vi "NI_FPGA_PPG.ProcCases.vi"(0 "i ref in":refnum<vi>, 1 "selector":string, 2 "Data":T1, 3 "call cluster":T2={"Object"="", "Selector"="", "CallType"=enum."synchronous", "Async Object"="", "Async Selector"="", "Data Descriptor"="", "Data"=[], "Error #"=0, "Expire"=0}, 5 "error in (no error)":errorcluster) -> (14 "i ref out":refnum<vi>, 17 "answer cluster":T2={"Object"="", "Selector"="", "CallType"=enum."synchronous", "Async Object"="", "Async Selector"="", "Data Descriptor"="", "Data"=[], "Error #"=0, "Expire"=0}, 19 "error out":errorcluster)   [LabVIEW 2014, in "NI_FPGA_PPG.lvlib"]
doc: "This method is called by a process from within the default case in the event loop. The methods of a class that are linked to events will be called from THIS method. Add your code here."
uses:
  NI_FPGA_PPG.lvlib
  CSCore/CSSystem/CoreDefs/CoreDefs.call_type.ctl
  CSCore/BaseProcess/BaseProcess.descriptor string definition.ctl
  CSCore/CSSystem/CoreDefs/CoreDefs.rawDataType.ctl
  CSCore/CSSystem/CoreLib/CoreLib.string 2 byte array.vi
  CSCore/CSSystem/CoreLib/CoreLib.int 2 byte array.vi
  CSCore/CSSystem/CoreLib/CoreLib.byte array 2 string.vi
  CSCore/CSSystem/CoreLib/CoreLib.byte array 2 int.vi
  CSCore/CSSystem/CoreLib/CoreLib.byte array 2 double.vi
  CSCore/CSSystem/CoreLib/CoreLib.lvlib
  CSCore/BaseProcess/BaseProcess.lvlib
  CSCore/CSApplicationBaseClasses/DeviceBase/DeviceBase.lvlib
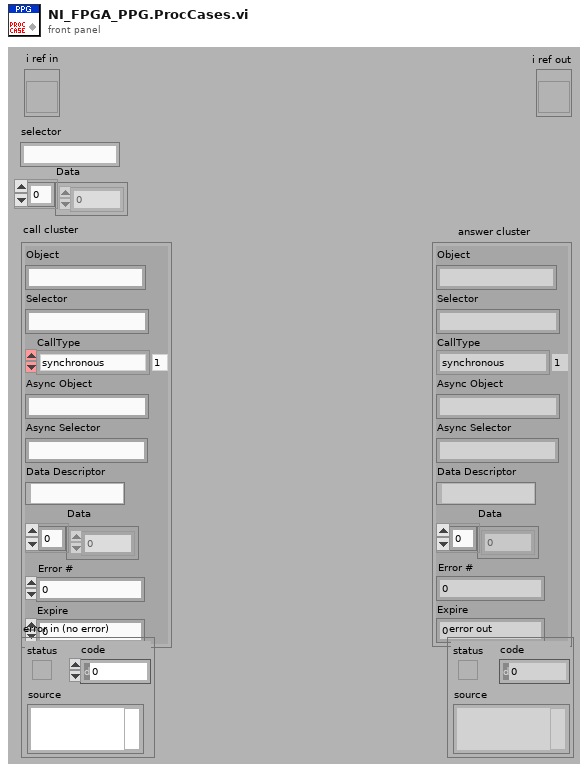
[diagram p1: front panel]
types:
  T1 = typedef "CoreDefs.rawDataType.ctl" = i8[]
  T2 = typedef "CoreDefs.call_type.ctl" = cluster{"Object":string, "Selector":string, "CallType":enum16{"simple", "synchronous", "asynchronous"}, "Async Object":string, "Async Selector":string, "Data Descriptor":T3, "Data":T1, "Error #":i32, "Expire":u32}
  T3 = typedef "BaseProcess.lvlib/BaseProcess.descriptor string definition.ctl" = string
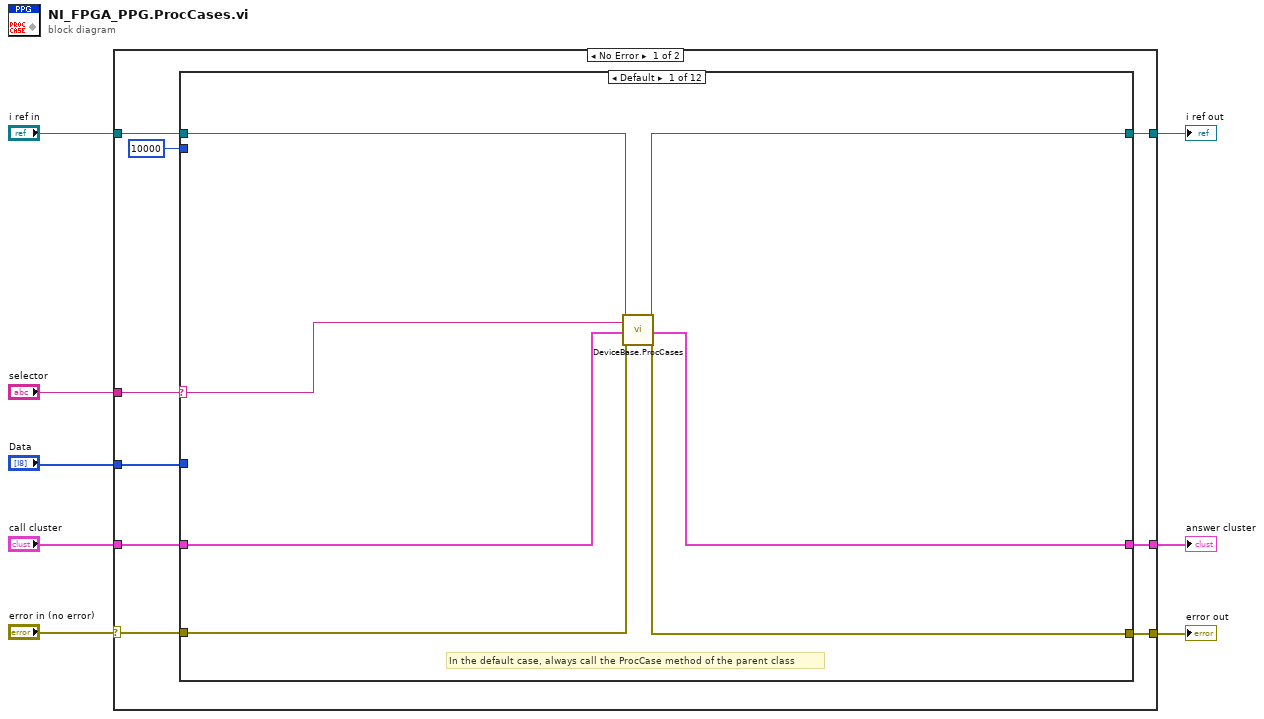
[diagram p0: block diagram]
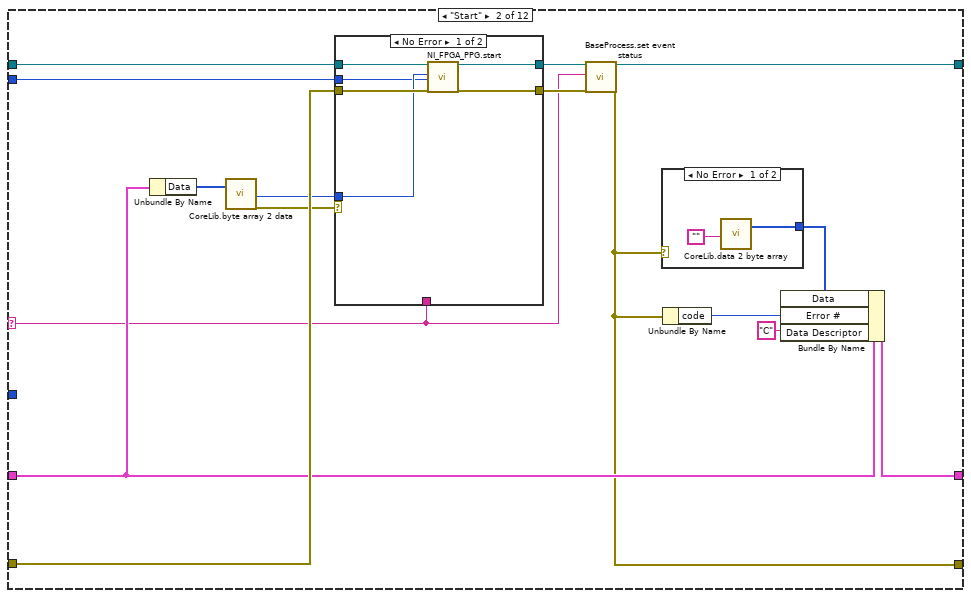
[diagram p2: hidden frame]
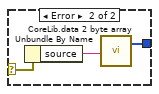
[diagram p3: hidden frame]
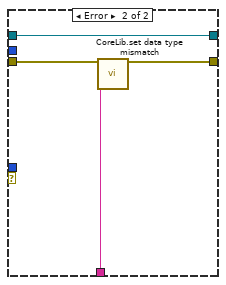
[diagram p4: hidden frame]
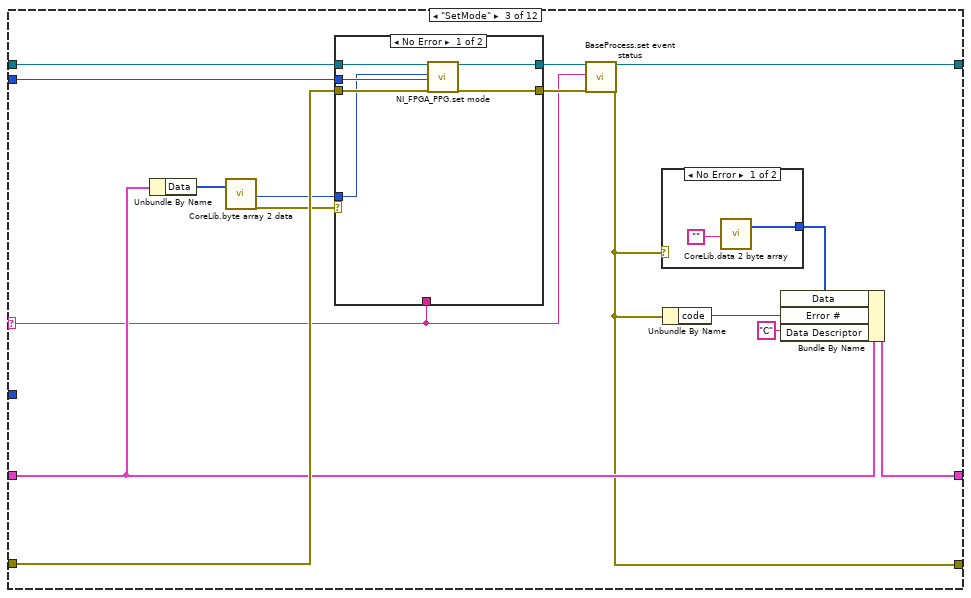
[diagram p5: hidden frame]
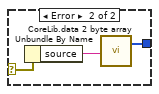
[diagram p6: hidden frame]
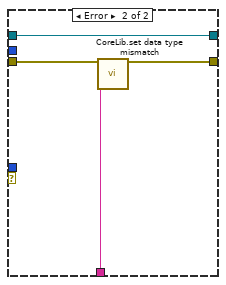
[diagram p7: hidden frame]
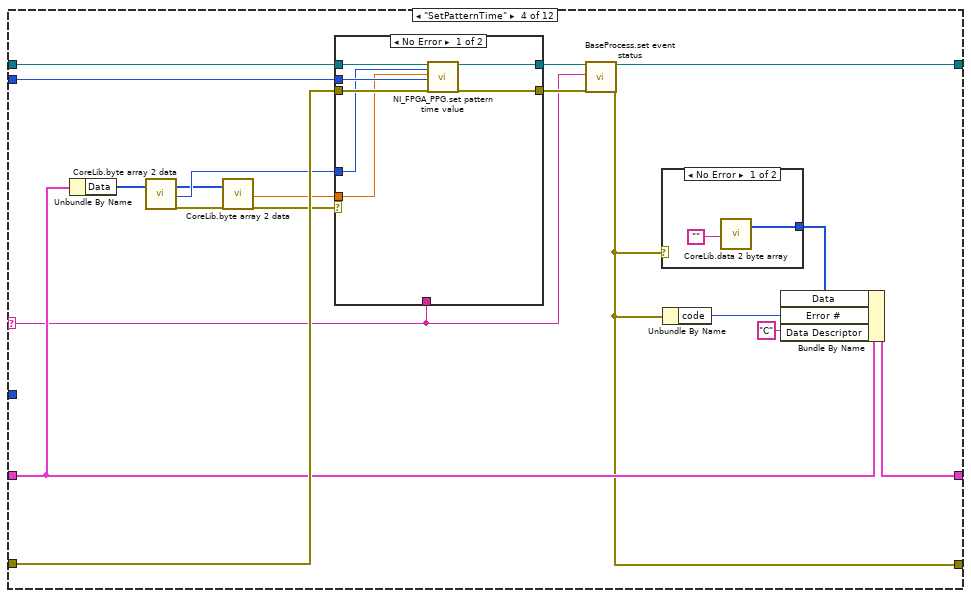
[diagram p8: hidden frame]
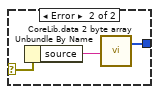
[diagram p9: hidden frame]
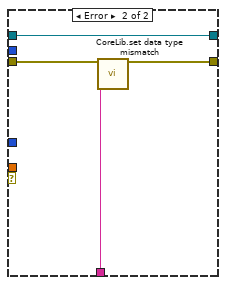
[diagram p10: hidden frame]
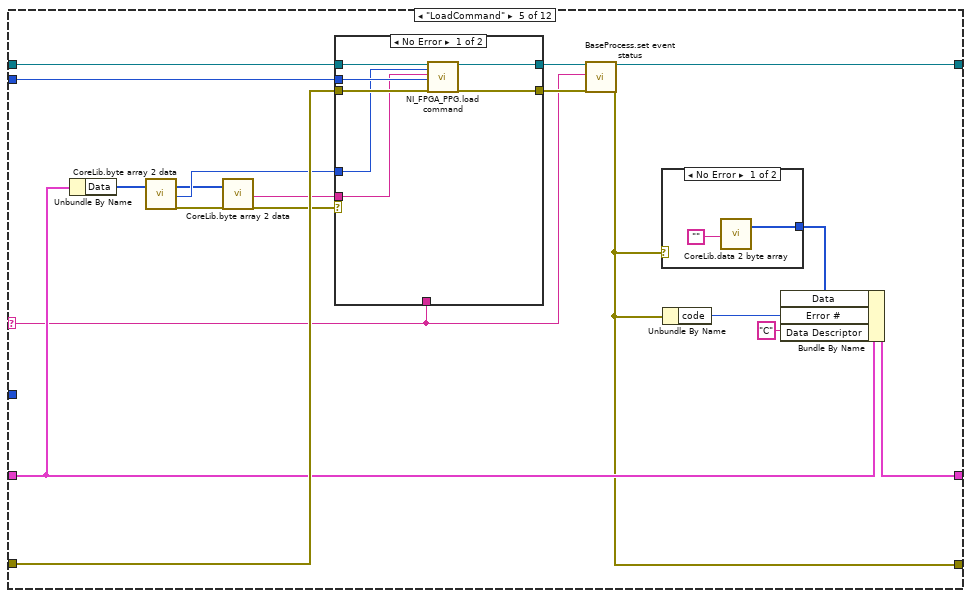
[diagram p11: hidden frame]
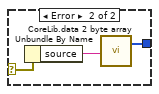
[diagram p12: hidden frame]
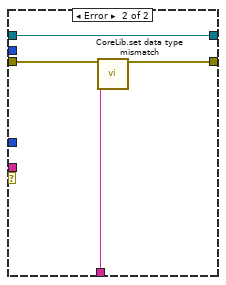
[diagram p13: hidden frame]
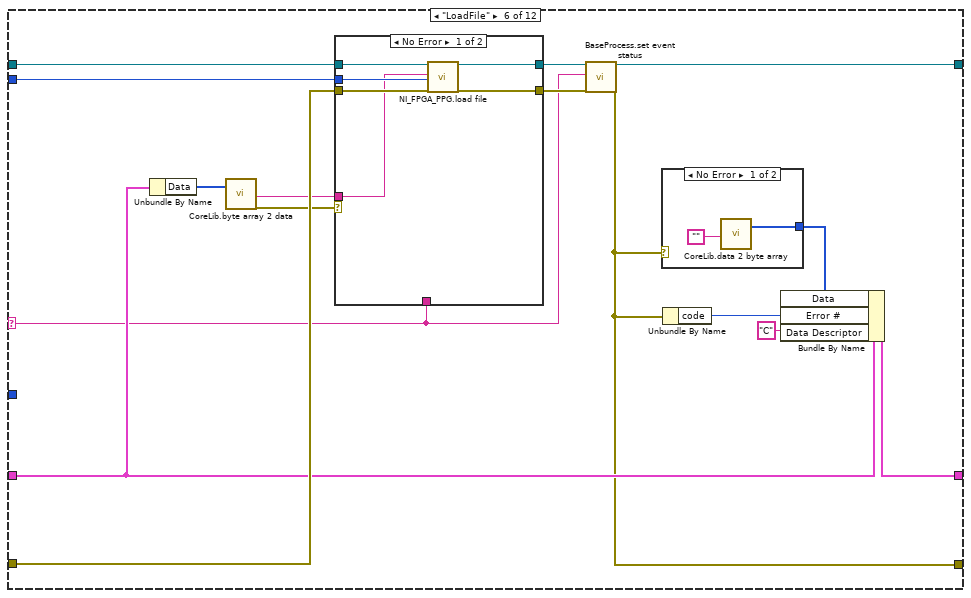
[diagram p14: hidden frame]
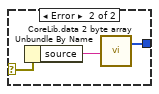
[diagram p15: hidden frame]
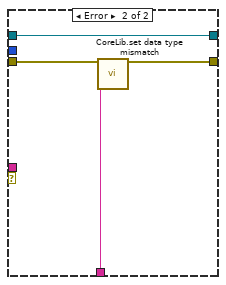
[diagram p16: hidden frame]
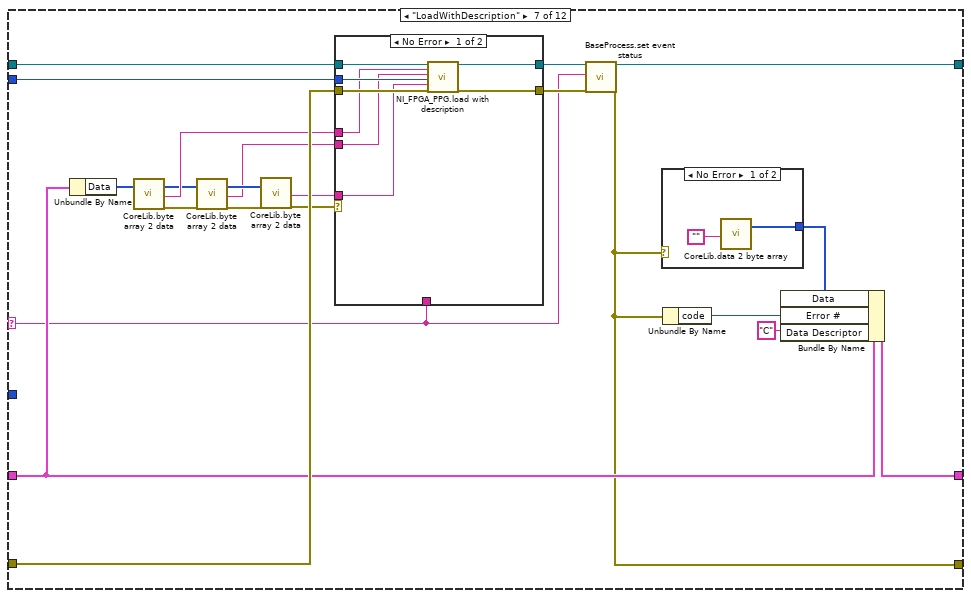
[diagram p17: hidden frame]
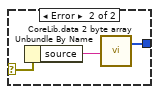
[diagram p18: hidden frame]
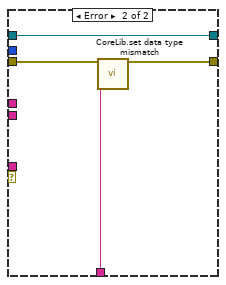
[diagram p19: hidden frame]
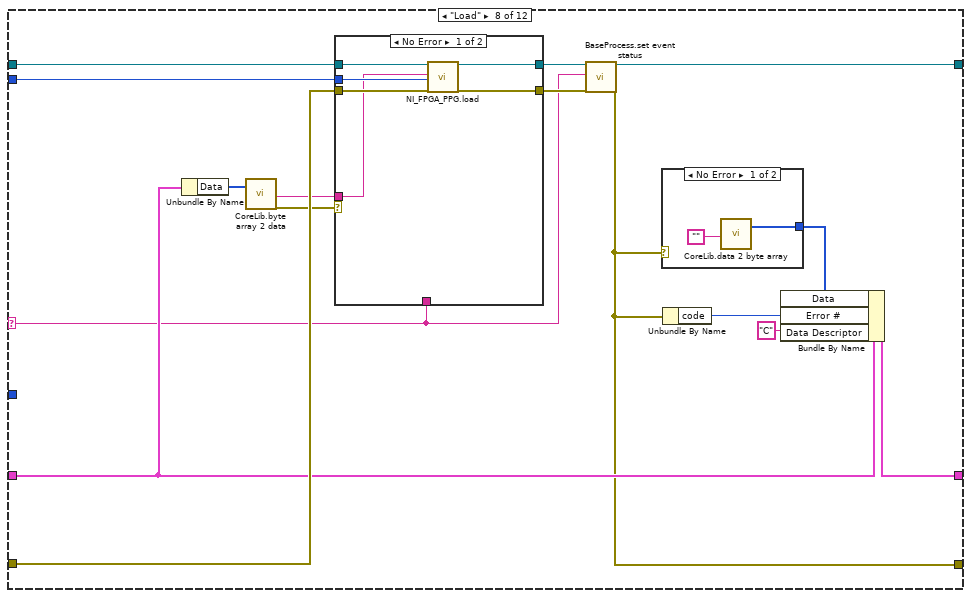
[diagram p20: hidden frame]
diagram:
  n1 = case shown="No Error" "error in (no error)" {
    selector: "error in (no error)" -> [w10 w331]
    tunnel: "selector" -> [w17 _]
    tunnel: [w16 w332] -> w7
    tunnel: "Data" -> [w15 _]
    tunnel: "call cluster" -> [w14 w332]
    tunnel: "i ref in" -> [w13 w333]
    tunnel: [w12 w333] -> w3
    tunnel: [w11 w331] -> w2
    frame No Error {
      n2 = case shown="Default" w17 {
        selector: w17 -> [w19 w31 w62 w96 w131 w163 w200 w233 w261 w279 w298 w316]
        tunnel: w15 -> [_ _ _ _ _ _ _ _ _ _ _ _]
        tunnel: w13 -> [w18 w40 w71 w105 w140 w172 w209 w242 w270 w288 w307 w325]
        tunnel: [w24 w30 w61 w95 w130 w162 w199 w232 w260 w278 w297 w315] -> w12
        tunnel: w14 -> [w20 w37 w68 w102 w137 w169 w206 w239 w267 w285 w304 w322]
        tunnel: [w21 w36 w67 w101 w136 w168 w205 w238 w266 w284 w303 w321] -> w16
        tunnel: w10 -> [w23 w39 w70 w104 w139 w171 w208 w241 w269 w287 w306 w324]
        tunnel: [w22 w32 w63 w97 w132 w164 w201 w234 w262 w280 w299 w317] -> w11
        tunnel: 10000 ("ms timeout") -> [_ w25 w56 w87 w122 w157 w188 w227 w258 w276 w295 w313]
        frame Default {
          # "In the default case, always call the ProcCase method of the parent class"
          n3 = call "DeviceBase.ProcCases.vi"("i ref in"=w18, "selector"=w19, "call cluster"=w20, "error in (no error)"=w23) -> ("i ref out"=w24:refnum<vi>, "answer cluster"=w21:T2, "error out"=w22:errorcluster)  [unwired: 13 in]
        }
        frame "Start" {
          n4 = Unbundle By Name(w37) -> ("Data"=w28:T1)
          n5 = call-poly "CoreLib.byte array 2 data.vi"("byteArray"=w28) -> ("i32"=w27:i32, "error out"=w26:errorcluster)  [unwired: 16 in, 1 out]
          n6 = case shown="No Error" w26 {
            tunnel: [w48 w55] -> w34
            tunnel: w40 -> [w51 w55]
            tunnel: w39 -> [w50 w54]
            tunnel: [w49 w53] -> w33
            tunnel: w31 -> [_ w52]
            tunnel: w27 -> [w47 _]
            tunnel: w25 -> [w46 _]
            frame No Error {
              n7 = call "NI_FPGA_PPG.start.vi"("i ref in"=w51, "start_addr"=w47, "ms timeout (10000)"=w46, "error in (no error)"=w50) -> ("i ref out"=w48:refnum<vi>, "error out"=w49:errorcluster)  [unwired: 13 in, 1 out]
            }
            frame Error {
              n8 = call "CoreLib.set data type mismatch.vi"("error in (no error)"=w54, "error source"=w52) -> ("error out"=w53:errorcluster)  [unwired: 17 in]
            }
          }
          n9 = call "BaseProcess.set event status.vi"("i ref in"=w34, "EventStatus"=w31, "error in (no error)"=w33) -> ("i ref out"=w30:refnum<vi>, "error out"=w32:errorcluster)  [unwired: 14 in, 1 out]
          n10 = case shown="No Error" w32 {
            selector: w32 -> [_ w45]
            tunnel: [w42 w44] -> w35
            frame No Error {
              n11 = call-poly "CoreLib.data 2 byte array.vi"("string"="" ("Empty String Constant")) -> ("byteArray out"=w42:T1)  [unwired: 18 in]
            }
            frame Error {
              n12 = Unbundle By Name(w45) -> ("source"=w43:string)
              n13 = call-poly "CoreLib.data 2 byte array.vi"("string"=w43) -> ("byteArray out"=w44:T1)  [unwired: 18 in]
            }
          }
          n14 = Unbundle By Name(w32) -> ("code"=w38:i32)
          n15 = Bundle By Name(cluster=w37, "Data"=w35, "Error #"=w38, "Data Descriptor"="C") -> (w36:T2)
        }
        frame "SetMode" {
          n16 = Unbundle By Name(w68) -> ("Data"=w59:T1)
          n17 = call-poly "CoreLib.byte array 2 data.vi"("byteArray"=w59) -> ("i32"=w58:i32, "error out"=w57:errorcluster)  [unwired: 16 in, 1 out]
          n18 = case shown="No Error" w57 {
            tunnel: [w79 w86] -> w65
            tunnel: w71 -> [w82 w86]
            tunnel: w70 -> [w81 w85]
            tunnel: [w80 w84] -> w64
            tunnel: w62 -> [_ w83]
            tunnel: w58 -> [w77 _]
            tunnel: w56 -> [w78 _]
            frame No Error {
              n19 = call "NI_FPGA_PPG.set mode.vi"("i ref in"=w82, "mode"=w77, "ms timeout (10000)"=w78, "error in (no error)"=w81) -> ("i ref out"=w79:refnum<vi>, "error out"=w80:errorcluster)  [unwired: 13 in, 1 out]
            }
            frame Error {
              n20 = call "CoreLib.set data type mismatch.vi"("error in (no error)"=w85, "error source"=w83) -> ("error out"=w84:errorcluster)  [unwired: 17 in]
            }
          }
          n21 = call "BaseProcess.set event status.vi"("i ref in"=w65, "EventStatus"=w62, "error in (no error)"=w64) -> ("i ref out"=w61:refnum<vi>, "error out"=w63:errorcluster)  [unwired: 14 in, 1 out]
          n22 = case shown="No Error" w63 {
            selector: w63 -> [_ w76]
            tunnel: [w73 w75] -> w66
            frame No Error {
              n23 = call-poly "CoreLib.data 2 byte array.vi"("string"="" ("Empty String Constant")) -> ("byteArray out"=w73:T1)  [unwired: 18 in]
            }
            frame Error {
              n24 = Unbundle By Name(w76) -> ("source"=w74:string)
              n25 = call-poly "CoreLib.data 2 byte array.vi"("string"=w74) -> ("byteArray out"=w75:T1)  [unwired: 18 in]
            }
          }
          n26 = Unbundle By Name(w63) -> ("code"=w69:i32)
          n27 = Bundle By Name(cluster=w68, "Data"=w66, "Error #"=w69, "Data Descriptor"="C") -> (w67:T2)
        }
        frame "SetPatternTime" {
          n28 = Unbundle By Name(w102) -> ("Data"=w93:T1)
          n29 = call-poly "CoreLib.byte array 2 data.vi"("byteArray"=w93) -> ("byteArray out"=w90:T1, "i32"=w92:i32, "error out"=w91:errorcluster)  [unwired: 16 in]
          n30 = call-poly "CoreLib.byte array 2 data.vi"("byteArray"=w90, "error in (no error)"=w91) -> ("d64"=w88:dbl, "error out"=w89:errorcluster)  [unwired: 15 in, 1 out]
          n31 = case shown="No Error" w89 {
            tunnel: [w114 w121] -> w99
            tunnel: w105 -> [w117 w121]
            tunnel: w104 -> [w116 w120]
            tunnel: [w115 w119] -> w98
            tunnel: w96 -> [_ w118]
            tunnel: w92 -> [w112 _]
            tunnel: w88 -> [w111 _]
            tunnel: w87 -> [w113 _]
            frame No Error {
              n32 = call "NI_FPGA_PPG.set pattern time value.vi"("i ref in"=w117, "memory_addr"=w112, "time [us]"=w111, "ms timeout (10000)"=w113, "error in (no error)"=w116) -> ("i ref out"=w114:refnum<vi>, "error out"=w115:errorcluster)  [unwired: 12 in, 1 out]
            }
            frame Error {
              n33 = call "CoreLib.set data type mismatch.vi"("error in (no error)"=w120, "error source"=w118) -> ("error out"=w119:errorcluster)  [unwired: 17 in]
            }
          }
          n34 = call "BaseProcess.set event status.vi"("i ref in"=w99, "EventStatus"=w96, "error in (no error)"=w98) -> ("i ref out"=w95:refnum<vi>, "error out"=w97:errorcluster)  [unwired: 14 in, 1 out]
          n35 = case shown="No Error" w97 {
            selector: w97 -> [_ w110]
            tunnel: [w107 w109] -> w100
            frame No Error {
              n36 = call-poly "CoreLib.data 2 byte array.vi"("string"="" ("Empty String Constant")) -> ("byteArray out"=w107:T1)  [unwired: 18 in]
            }
            frame Error {
              n37 = Unbundle By Name(w110) -> ("source"=w108:string)
              n38 = call-poly "CoreLib.data 2 byte array.vi"("string"=w108) -> ("byteArray out"=w109:T1)  [unwired: 18 in]
            }
          }
          n39 = Unbundle By Name(w97) -> ("code"=w103:i32)
          n40 = Bundle By Name(cluster=w102, "Data"=w100, "Error #"=w103, "Data Descriptor"="C") -> (w101:T2)
        }
        frame "LoadCommand" {
          n41 = Unbundle By Name(w137) -> ("Data"=w128:T1)
          n42 = call-poly "CoreLib.byte array 2 data.vi"("byteArray"=w128) -> ("byteArray out"=w125:T1, "i32"=w127:i32, "error out"=w126:errorcluster)  [unwired: 16 in]
          n43 = call-poly "CoreLib.byte array 2 data.vi"("byteArray"=w125, "error in (no error)"=w126) -> ("string"=w123:string, "error out"=w124:errorcluster)  [unwired: 15 in, 1 out]
          n44 = case shown="No Error" w124 {
            tunnel: [w149 w156] -> w134
            tunnel: w140 -> [w152 w156]
            tunnel: w139 -> [w151 w155]
            tunnel: [w150 w154] -> w133
            tunnel: w131 -> [_ w153]
            tunnel: w127 -> [w147 _]
            tunnel: w123 -> [w146 _]
            tunnel: w122 -> [w148 _]
            frame No Error {
              n45 = call "NI_FPGA_PPG.load command.vi"("i ref in"=w152, "mem_addr"=w147, "command"=w146, "ms timeout (10000)"=w148, "error in (no error)"=w151) -> ("i ref out"=w149:refnum<vi>, "error out"=w150:errorcluster)  [unwired: 12 in, 1 out]
            }
            frame Error {
              n46 = call "CoreLib.set data type mismatch.vi"("error in (no error)"=w155, "error source"=w153) -> ("error out"=w154:errorcluster)  [unwired: 17 in]
            }
          }
          n47 = call "BaseProcess.set event status.vi"("i ref in"=w134, "EventStatus"=w131, "error in (no error)"=w133) -> ("i ref out"=w130:refnum<vi>, "error out"=w132:errorcluster)  [unwired: 14 in, 1 out]
          n48 = case shown="No Error" w132 {
            selector: w132 -> [_ w145]
            tunnel: [w142 w144] -> w135
            frame No Error {
              n49 = call-poly "CoreLib.data 2 byte array.vi"("string"="" ("Empty String Constant")) -> ("byteArray out"=w142:T1)  [unwired: 18 in]
            }
            frame Error {
              n50 = Unbundle By Name(w145) -> ("source"=w143:string)
              n51 = call-poly "CoreLib.data 2 byte array.vi"("string"=w143) -> ("byteArray out"=w144:T1)  [unwired: 18 in]
            }
          }
          n52 = Unbundle By Name(w132) -> ("code"=w138:i32)
          n53 = Bundle By Name(cluster=w137, "Data"=w135, "Error #"=w138, "Data Descriptor"="C") -> (w136:T2)
        }
        frame "LoadFile" {
          n54 = Unbundle By Name(w169) -> ("Data"=w160:T1)
          n55 = call-poly "CoreLib.byte array 2 data.vi"("byteArray"=w160) -> ("string"=w159:string, "error out"=w158:errorcluster)  [unwired: 16 in, 1 out]
          n56 = case shown="No Error" w158 {
            tunnel: [w180 w187] -> w166
            tunnel: w172 -> [w183 w187]
            tunnel: w171 -> [w182 w186]
            tunnel: [w181 w185] -> w165
            tunnel: w163 -> [_ w184]
            tunnel: w159 -> [w178 _]
            tunnel: w157 -> [w179 _]
            frame No Error {
              n57 = call "NI_FPGA_PPG.load file.vi"("i ref in"=w183, "file"=w178, "ms timeout (10000)"=w179, "error in (no error)"=w182) -> ("i ref out"=w180:refnum<vi>, "error out"=w181:errorcluster)  [unwired: 13 in, 1 out]
            }
            frame Error {
              n58 = call "CoreLib.set data type mismatch.vi"("error in (no error)"=w186, "error source"=w184) -> ("error out"=w185:errorcluster)  [unwired: 17 in]
            }
          }
          n59 = call "BaseProcess.set event status.vi"("i ref in"=w166, "EventStatus"=w163, "error in (no error)"=w165) -> ("i ref out"=w162:refnum<vi>, "error out"=w164:errorcluster)  [unwired: 14 in, 1 out]
          n60 = case shown="No Error" w164 {
            selector: w164 -> [_ w177]
            tunnel: [w174 w176] -> w167
            frame No Error {
              n61 = call-poly "CoreLib.data 2 byte array.vi"("string"="" ("Empty String Constant")) -> ("byteArray out"=w174:T1)  [unwired: 18 in]
            }
            frame Error {
              n62 = Unbundle By Name(w177) -> ("source"=w175:string)
              n63 = call-poly "CoreLib.data 2 byte array.vi"("string"=w175) -> ("byteArray out"=w176:T1)  [unwired: 18 in]
            }
          }
          n64 = Unbundle By Name(w164) -> ("code"=w170:i32)
          n65 = Bundle By Name(cluster=w169, "Data"=w167, "Error #"=w170, "Data Descriptor"="C") -> (w168:T2)
        }
        frame "LoadWithDescription" {
          n66 = Unbundle By Name(w206) -> ("Data"=w197:T1)
          n67 = call-poly "CoreLib.byte array 2 data.vi"("byteArray"=w197) -> ("byteArray out"=w192:T1, "string"=w196:string, "error out"=w193:errorcluster)  [unwired: 16 in]
          n68 = call-poly "CoreLib.byte array 2 data.vi"("byteArray"=w192, "error in (no error)"=w193) -> ("byteArray out"=w195:T1, "string"=w191:string, "error out"=w194:errorcluster)  [unwired: 15 in]
          n69 = call-poly "CoreLib.byte array 2 data.vi"("byteArray"=w195, "error in (no error)"=w194) -> ("string"=w189:string, "error out"=w190:errorcluster)  [unwired: 15 in, 1 out]
          n70 = case shown="No Error" w190 {
            tunnel: [w219 w226] -> w203
            tunnel: w209 -> [w222 w226]
            tunnel: w208 -> [w221 w225]
            tunnel: [w220 w224] -> w202
            tunnel: w200 -> [_ w223]
            tunnel: w196 -> [w217 _]
            tunnel: w191 -> [w216 _]
            tunnel: w189 -> [w215 _]
            tunnel: w188 -> [w218 _]
            frame No Error {
              n71 = call "NI_FPGA_PPG.load with description.vi"("i ref in"=w222, "cmd_data_string"=w217, "cmd_data_description_string"=w216, "ms timeout (10000)"=w218, "channel_description_string"=w215, "error in (no error)"=w221) -> ("i ref out"=w219:refnum<vi>, "error out"=w220:errorcluster)  [unwired: 11 in, 1 out]
            }
            frame Error {
              n72 = call "CoreLib.set data type mismatch.vi"("error in (no error)"=w225, "error source"=w223) -> ("error out"=w224:errorcluster)  [unwired: 17 in]
            }
          }
          n73 = call "BaseProcess.set event status.vi"("i ref in"=w203, "EventStatus"=w200, "error in (no error)"=w202) -> ("i ref out"=w199:refnum<vi>, "error out"=w201:errorcluster)  [unwired: 14 in, 1 out]
          n74 = case shown="No Error" w201 {
            selector: w201 -> [_ w214]
            tunnel: [w211 w213] -> w204
            frame No Error {
              n75 = call-poly "CoreLib.data 2 byte array.vi"("string"="" ("Empty String Constant")) -> ("byteArray out"=w211:T1)  [unwired: 18 in]
            }
            frame Error {
              n76 = Unbundle By Name(w214) -> ("source"=w212:string)
              n77 = call-poly "CoreLib.data 2 byte array.vi"("string"=w212) -> ("byteArray out"=w213:T1)  [unwired: 18 in]
            }
          }
          n78 = Unbundle By Name(w201) -> ("code"=w207:i32)
          n79 = Bundle By Name(cluster=w206, "Data"=w204, "Error #"=w207, "Data Descriptor"="C") -> (w205:T2)
        }
        frame "Load" {
          n80 = Unbundle By Name(w239) -> ("Data"=w230:T1)
          n81 = call-poly "CoreLib.byte array 2 data.vi"("byteArray"=w230) -> ("string"=w229:string, "error out"=w228:errorcluster)  [unwired: 16 in, 1 out]
          n82 = case shown="No Error" w228 {
            tunnel: [w250 w257] -> w236
            tunnel: w242 -> [w253 w257]
            tunnel: w241 -> [w252 w256]
            tunnel: [w251 w255] -> w235
            tunnel: w233 -> [_ w254]
            tunnel: w229 -> [w248 _]
            tunnel: w227 -> [w249 _]
            frame No Error {
              n83 = call "NI_FPGA_PPG.load.vi"("i ref in"=w253, "cmd_data_string"=w248, "ms timeout (10000)"=w249, "error in (no error)"=w252) -> ("i ref out"=w250:refnum<vi>, "error out"=w251:errorcluster)  [unwired: 13 in, 1 out]
            }
            frame Error {
              n84 = call "CoreLib.set data type mismatch.vi"("error in (no error)"=w256, "error source"=w254) -> ("error out"=w255:errorcluster)  [unwired: 17 in]
            }
          }
          n85 = call "BaseProcess.set event status.vi"("i ref in"=w236, "EventStatus"=w233, "error in (no error)"=w235) -> ("i ref out"=w232:refnum<vi>, "error out"=w234:errorcluster)  [unwired: 14 in, 1 out]
          n86 = case shown="No Error" w234 {
            selector: w234 -> [_ w247]
            tunnel: [w244 w246] -> w237
            frame No Error {
              n87 = call-poly "CoreLib.data 2 byte array.vi"("string"="" ("Empty String Constant")) -> ("byteArray out"=w244:T1)  [unwired: 18 in]
            }
            frame Error {
              n88 = Unbundle By Name(w247) -> ("source"=w245:string)
              n89 = call-poly "CoreLib.data 2 byte array.vi"("string"=w245) -> ("byteArray out"=w246:T1)  [unwired: 18 in]
            }
          }
          n90 = Unbundle By Name(w234) -> ("code"=w240:i32)
          n91 = Bundle By Name(cluster=w239, "Data"=w237, "Error #"=w240, "Data Descriptor"="C") -> (w238:T2)
        }
        frame "Stop" {
          n92 = call "NI_FPGA_PPG.stop.vi"("i ref in"=w270, "ms timeout (10000)"=w258, "error in (no error)"=w269) -> ("i ref out"=w264:refnum<vi>, "error out"=w263:errorcluster)  [unwired: 13 in, 2 out]
          n93 = call "BaseProcess.set event status.vi"("i ref in"=w264, "EventStatus"=w261, "error in (no error)"=w263) -> ("i ref out"=w260:refnum<vi>, "error out"=w262:errorcluster)  [unwired: 14 in, 1 out]
          n94 = case shown="No Error" w262 {
            selector: w262 -> [_ w274]
            tunnel: [w271 w273] -> w265
            frame No Error {
              n95 = call-poly "CoreLib.data 2 byte array.vi"() -> ("byteArray out"=w271:T1)  [unwired: 19 in]
            }
            frame Error {
              n96 = Unbundle By Name(w274) -> ("source"=w272:string)
              n97 = call-poly "CoreLib.data 2 byte array.vi"("string"=w272) -> ("byteArray out"=w273:T1)  [unwired: 18 in]
            }
          }
          n98 = Unbundle By Name(w262) -> ("code"=w268:i32)
          n99 = Bundle By Name(cluster=w267, "Data"=w265, "Error #"=w268, "Data Descriptor"="I:1") -> (w266:T2)
        }
        frame "GetStatus" {
          n100 = call "NI_FPGA_PPG.get status.vi"("i ref in"=w288, "ms timeout (10000)"=w276, "error in (no error)"=w287) -> ("i ref out"=w282:refnum<vi>, "FPGA_status"=w275:i32, "error out"=w281:errorcluster)  [unwired: 13 in, 1 out]
          n101 = call "BaseProcess.set event status.vi"("i ref in"=w282, "EventStatus"=w279, "error in (no error)"=w281) -> ("i ref out"=w278:refnum<vi>, "error out"=w280:errorcluster)  [unwired: 14 in, 1 out]
          n102 = case shown="No Error" w280 {
            selector: w280 -> [_ w293]
            tunnel: [w290 w292] -> w283
            tunnel: w275 -> [w289 _]
            frame No Error {
              n103 = call-poly "CoreLib.data 2 byte array.vi"("i32"=w289) -> ("byteArray out"=w290:T1)  [unwired: 18 in]
            }
            frame Error {
              n104 = Unbundle By Name(w293) -> ("source"=w291:string)
              n105 = call-poly "CoreLib.data 2 byte array.vi"("string"=w291) -> ("byteArray out"=w292:T1)  [unwired: 18 in]
            }
          }
          n106 = Unbundle By Name(w280) -> ("code"=w286:i32)
          n107 = Bundle By Name(cluster=w285, "Data"=w283, "Error #"=w286, "Data Descriptor"="I:1") -> (w284:T2)
        }
        frame "GetMode" {
          n108 = call "NI_FPGA_PPG.get mode.vi"("i ref in"=w307, "ms timeout (10000)"=w295, "error in (no error)"=w306) -> ("i ref out"=w301:refnum<vi>, "mode"=w294:i32, "error out"=w300:errorcluster)  [unwired: 13 in, 1 out]
          n109 = call "BaseProcess.set event status.vi"("i ref in"=w301, "EventStatus"=w298, "error in (no error)"=w300) -> ("i ref out"=w297:refnum<vi>, "error out"=w299:errorcluster)  [unwired: 14 in, 1 out]
          n110 = case shown="No Error" w299 {
            selector: w299 -> [_ w312]
            tunnel: [w309 w311] -> w302
            tunnel: w294 -> [w308 _]
            frame No Error {
              n111 = call-poly "CoreLib.data 2 byte array.vi"("i32"=w308) -> ("byteArray out"=w309:T1)  [unwired: 18 in]
            }
            frame Error {
              n112 = Unbundle By Name(w312) -> ("source"=w310:string)
              n113 = call-poly "CoreLib.data 2 byte array.vi"("string"=w310) -> ("byteArray out"=w311:T1)  [unwired: 18 in]
            }
          }
          n114 = Unbundle By Name(w299) -> ("code"=w305:i32)
          n115 = Bundle By Name(cluster=w304, "Data"=w302, "Error #"=w305, "Data Descriptor"="I:1") -> (w303:T2)
        }
        frame "Reset" {
          n116 = call "NI_FPGA_PPG.reset.vi"("i ref in"=w325, "ms timeout (10000)"=w313, "error in (no error)"=w324) -> ("i ref out"=w319:refnum<vi>, "error out"=w318:errorcluster)  [unwired: 14 in, 1 out]
          n117 = call "BaseProcess.set event status.vi"("i ref in"=w319, "EventStatus"=w316, "error in (no error)"=w318) -> ("i ref out"=w315:refnum<vi>, "error out"=w317:errorcluster)  [unwired: 14 in, 1 out]
          n118 = case shown="No Error" w317 {
            selector: w317 -> [_ w330]
            tunnel: [w327 w329] -> w320
            frame No Error {
              n119 = call-poly "CoreLib.data 2 byte array.vi"("string"="" ("Empty String Constant")) -> ("byteArray out"=w327:T1)  [unwired: 18 in]
            }
            frame Error {
              n120 = Unbundle By Name(w330) -> ("source"=w328:string)
              n121 = call-poly "CoreLib.data 2 byte array.vi"("string"=w328) -> ("byteArray out"=w329:T1)  [unwired: 18 in]
            }
          }
          n122 = Unbundle By Name(w317) -> ("code"=w323:i32)
          n123 = Bundle By Name(cluster=w322, "Data"=w320, "Error #"=w323, "Data Descriptor"="C") -> (w321:T2)
        }
      }
    }
    frame Error {
    }
  }
  "answer cluster" <- w7
  "i ref out" <- w3
  "error out" <- w2
